vi "Test and Log Effeciency.vi"(4 "Power Out":dbl, 6 "Power In":dbl, 7 "Position":u32, 10 "Test Voltage":string, 11 "Efficiency Test":refnum<class "Efficiency Test.lvclass">) -> (3 "Result":bool)   [LabVIEW 2015, in "Efficiency Test.lvclass"]
uses:
  Efficiency Test.lvclass
  Test Class/Test Class.lvclass
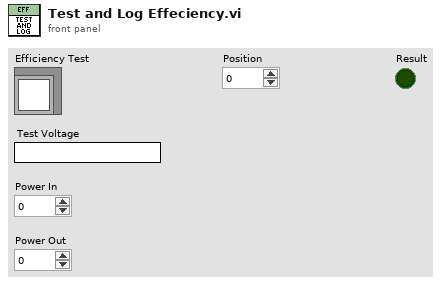
[diagram p1: front panel]
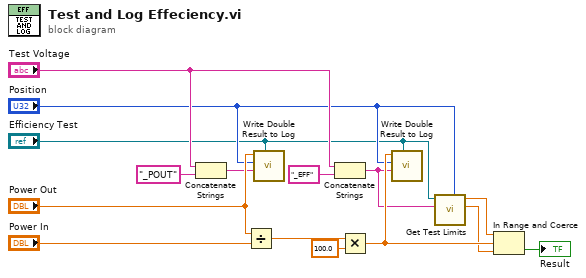
[diagram p0: block diagram]
diagram:
  n1 = Concatenate Strings("Test Voltage", "_POUT" ("string")) -> (w6:string)
  n2 = Divide(x="Power Out", y="Power In") -> (x/y=w15:dbl)
  n3 = call "Write Double Result to Log.vi"("Test Class in"="Efficiency Test", "Label"=w6, "Position"="Position", "Value"="Power Out") -> ()  [unwired: 7 in, 1 out]
  n4 = Concatenate Strings("Test Voltage", "_EFF" ("string")) -> (w1:string)
  n5 = Multiply(x=w15, y=100.0) -> (x*y=w8:dbl)
  n6 = call "Write Double Result to Log.vi"("Test Class in"="Efficiency Test", "Label"=w1, "Position"="Position", "Value"=w8) -> ()  [unwired: 7 in, 1 out]
  n7 = call "Get Test Limits.vi"("Position"="Position", "Channel"=w1, "Test Class in"="Efficiency Test") -> ("Lower Limit"=w4:dbl, "Upper Limit"=w5:dbl)  [unwired: 6 in, 1 out]
  n8 = In Range and Coerce(upper limit=w5, x=w8, lower limit=w4) -> (In Range?=→"Result":bool)  [unwired: 1 out]
